vi "Update Mode Menu Items.vi"(8 "error in (no error)":errorcluster, 11 "PS Control Actor in":refnum<class "PS Control Actor.lvclass">) -> (0 "error out":errorcluster, 3 "PS Control Actor out":refnum<class "PS Control Actor.lvclass">)   [LabVIEW 2019, in "PS Control Actor.lvlib" / "PS Control Actor.lvclass"]
uses:
  PS Control Actor.lvclass
  <vilib>/Utility/miscctls.llb/LVStringsAndValuesArrayTypeDef_U16.ctl
  PS Control Actor.lvclass/PS Control Actor.ctl
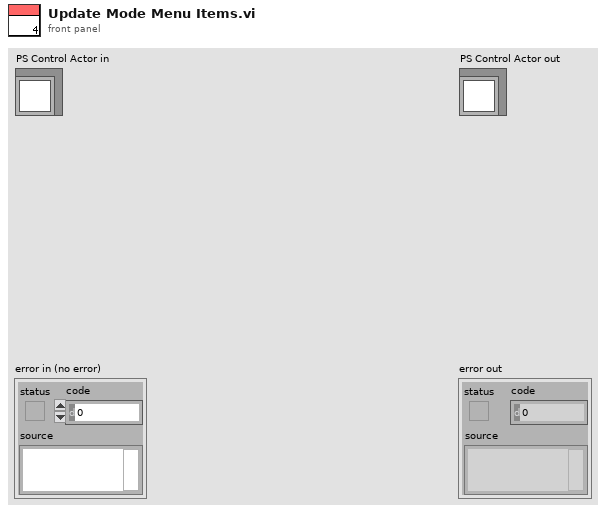
[diagram p1: front panel]
types:
  T1 = typedef "LVStringsAndValuesArrayTypeDef_U16.ctl" = cluster{"String":string, "Value":u16}[]
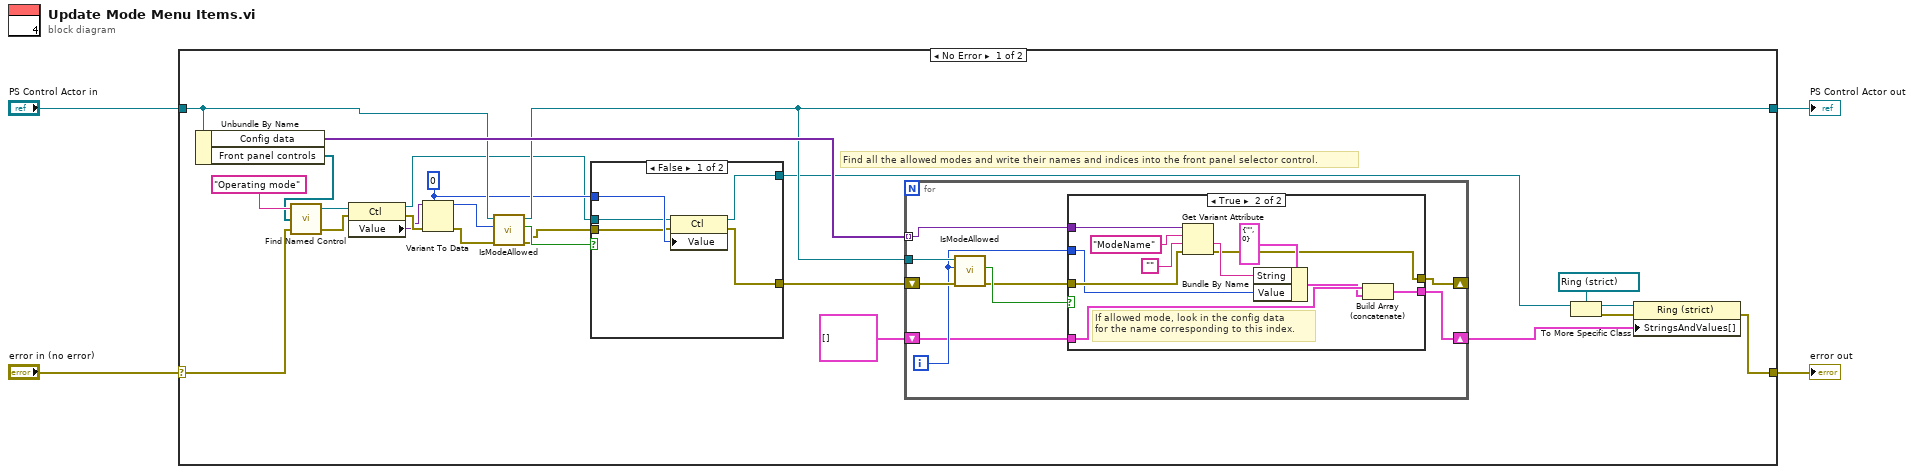
[diagram p0: block diagram]
diagram:
  n1 = case shown="No Error" "error in (no error)" {
    selector: "error in (no error)" -> [w19 w59]
    tunnel: [w21 w59] -> w3
    tunnel: [w11 w58] -> w1
    tunnel: "PS Control Actor in" -> [w13 w58]
    frame No Error {
      w9 = u16 0
      # "Find all the allowed modes and write their names and indices into the front panel selector control."
      n2 = Unbundle By Name(w13) -> ("Config data"=w28:variant[], "Front panel controls"=w20:refnum<vi>[])
      n3 = call "Find Named Control.vi"("error in"=w19, "All Controls"=w20, "Control Name"="Operating mode") -> ("error out"=w17:errorcluster, "Ctl Refnum"=w18:refnum<vi>)  [unwired: 1 out]
      n4 = property class="Ctl"(reference=w18, error in=w17) -> (reference out=w8:refnum<vi>, error out=w16:errorcluster, "Value"=w15:variant)
      n5 = Variant To Data(error in=w16, type=w9, Variant=w15) -> (data=w12:u16, error out=w14:errorcluster)
      n6 = call "IsModeAllowed.vi"("error in (no error)"=w14, "Mode"=w12, "PS Control Actor in"=w13) -> ("error out"=w7:errorcluster, "Allowed"=w10:bool, "PS Control Actor out"=w11:refnum<class "PS Control Actor.lvclass">)  [unwired: 6 in]
      n7 = case shown="False" w10 {
        tunnel: w9 -> [w33 _]
        tunnel: w8 -> [w32 w35]
        tunnel: w7 -> [w31 w34]
        tunnel: [w30 w34] -> w6
        tunnel: [w29 w35] -> w5
        frame False {
          n8 = property class="Ctl"(reference=w32, error in=w31, "Value"=w33) -> (reference out=w29:refnum<vi>, error out=w30:errorcluster)
        }
        frame True {
        }
      }
      n9 = for {
        tunnel: w28 -> [w40] mode=indexing
        tunnel: w11 -> [w43]
        shift-right: [w37] -> w23
        shift-left: T1 [] ("Strings And Values []") -> [w38]
        shift-right: [w36] -> _
        shift-left: w6 -> [w44]
        i -> [w41]
        n10 = call "IsModeAllowed.vi"("error in (no error)"=w44, "Mode"=w41, "PS Control Actor in"=w43) -> ("error out"=w39:errorcluster, "Allowed"=w42:bool)  [unwired: 6 in, 1 out]
        n11 = case shown="True" w42 {
          tunnel: w41 -> [_ w51]
          tunnel: w40 -> [_ w56]
          tunnel: w39 -> [w45 w54]
          tunnel: w38 -> [w46 w50]
          tunnel: [w46 w48] -> w37
          tunnel: [w45 w47] -> w36
          frame False {
          }
          frame True {
            # "If allowed mode, look in the config data\nfor the name corresponding to this index."
            n12 = Get Variant Attribute(Variant=w56, name="ModeName", default value (empty Variant)="", error in=w54) -> (value=w52:string, error out=w47:errorcluster)  [unwired: 2 out]
            n13 = Bundle By Name(cluster=cluster{"String":string, "Value":u16} {"String"="", "Value"=0}, "String"=w52, "Value"=w51) -> (w49:cluster{"String":string, "Value":u16})
            n14 = Build Array (concatenate)(w50, w49) -> (w48:T1)
          }
        }
      }
      n15 = To More Specific Class(target class=refnum<vi> refnum ("Ring"), reference=w5) -> (specific class reference=w27:refnum<vi>, error out=w22:errorcluster)  [unwired: 1 in]
      n16 = property class="Ring (strict)"(reference=w27, error in=w22, "StringsAndValues[]"=w23) -> (error out=w21:errorcluster)  [unwired: 1 out]
    }
    frame Error {
    }
  }
  "error out" <- w3
  "PS Control Actor out" <- w1
